vi "pcap dump.vi"(6 "len (0)":u32, 8 "error in":errorcluster, 9 "timeval":T1, 10 "Packet in":u8[](array[numeric]), 11 "pcap_dumper_t in":u64) -> (0 "error out":errorcluster, 3 "pcap_dumper_t out":u64)   [LabVIEW 2020, in "libpcaplv.lvlib"]
uses:
  libpcaplv.lvlib
  _typedefs/timeval_type_x64.ctl
  _typedefs/pcap_pkthdr_type_x86.ctl
  _typedefs/timeval_type_x86.ctl
  <vilib>/Utility/sysdir.llb/Get System Directory.vi
  _typedefs/pcap_pkthdr_type_x64.ctl
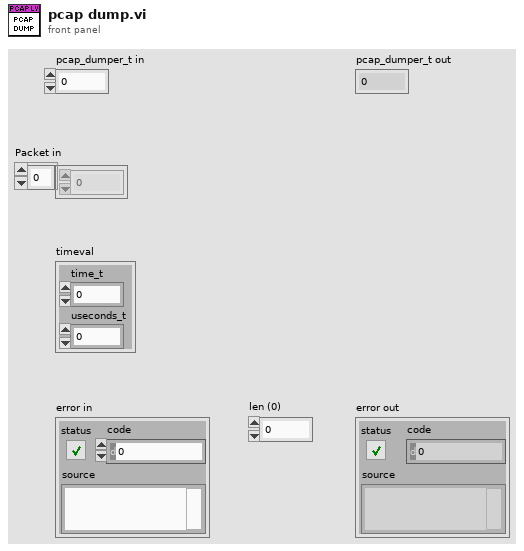
[diagram p1: front panel]
types:
  T1 = typedef "libpcaplv.lvlib/timeval_type_x64.ctl" = cluster{"time_t":u64, "useconds_t":u64}
  T2 = typedef "libpcaplv.lvlib/pcap_pkthdr_type_x64.ctl" = cluster{"timeval":T1, "caplen":u32, "len":u32}
  T3 = typedef "libpcaplv.lvlib/pcap_pkthdr_type_x86.ctl" = cluster{"timeval":T4, "caplen":u32, "len":u32}
  T4 = typedef "libpcaplv.lvlib/timeval_type_x86.ctl" = cluster{"time_t":u32, "useconds_t":u32}
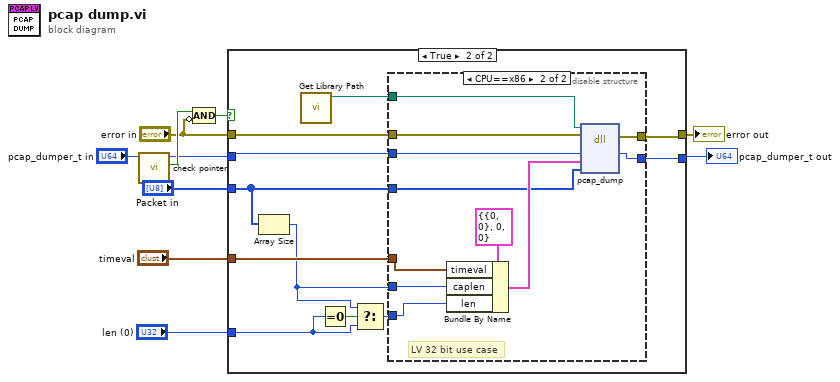
[diagram p0: block diagram]
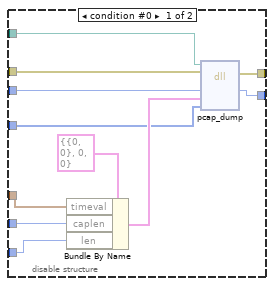
[diagram p3: hidden frame]
diagram:
  n1 = call "check pointer.vi"("pointer in"="pcap_dumper_t in") -> ("ok"=w9:bool, "pointer out"=w7:u64)  [unwired: 9 in]
  n2 = Compound Arithmetic op=AND(w9, invert "error in") -> (w6:bool)
  n3 = case shown="True" w6 {
    tunnel: [w11 w20] -> w10
    tunnel: w7 -> [w12 w22]
    tunnel: "error in" -> [w11 w23]
    tunnel: [w12 w21] -> w4
    tunnel: "Packet in" -> [_ w18]
    tunnel: "len (0)" -> [_ w14]
    tunnel: "timeval" -> [_ w19]
    frame False {
    }
    frame True {
      n4 = Array Size(array=w18) -> (size(s)=w17:i32)
      n5 = call "Get Library Path.vi"() -> ("library path"=w13:path)  [unwired: 11 in]
      n6 = Equal To 0?(x=w14) -> (x = 0?=w15:bool)
      n7 = Select(t=w17, s=w15, f=w14) -> (s? t:f=w16:u32)
      n8 = disable-structure shown="CPU==x86" {
        disable-tunnel: w23 -> [w34 w45]
        disable-tunnel: w22 -> [w33 w44]
        disable-tunnel: [w32 w43] -> w21
        disable-tunnel: [w31 w42] -> w20
        disable-tunnel: w19 -> [w28 w39]
        disable-tunnel: w18 -> [w27 w38]
        disable-tunnel: w17 -> [w26 w37]
        disable-tunnel: w16 -> [w25 w36]
        disable-tunnel: w13 -> [w24 w35]
        frame condition #0 {
          n9 = Bundle By Name(cluster=T2 {"timeval"={"time_t"=0, "useconds_t"=0}, "caplen"=0, "len"=0}, "timeval"=w28, "caplen"=w26, "len"=w25) -> (w29:T2)
          n10 = dll-call lib="libpcap.*" fn="pcap_dump"(path in=w24, error in=w34, "pcap_dumper_t"=w33, "pcap_hdr"=w29, "sp"=w27) -> (error out=w31:errorcluster, "pcap_dumper_t"=w32:u64)  [unwired: 4 in, 1 out]
        }
        frame condition #1 (active) {
          # "LV 32 bit use case"
          n11 = Bundle By Name(cluster=T3 {"timeval"={"time_t"=0, "useconds_t"=0}, "caplen"=0, "len"=0}, "timeval"=w39, "caplen"=w37, "len"=w36) -> (w40:T3)
          n12 = dll-call lib="libpcap.*" fn="pcap_dump"(path in=w35, error in=w45, "pcap_dumper_t"=w44, "pcap_hdr"=w40, "sp"=w38) -> (error out=w42:errorcluster, "pcap_dumper_t"=w43:u64)  [unwired: 4 in, 1 out]
        }
      }
    }
  }
  "pcap_dumper_t out" <- w4
  "error out" <- w10
